vi "Testing.vi"() -> ()   [LabVIEW 2013]
panel:
  in  "Image Name":string="Test1"
  in  "File Name":string="Checkout1"
  out "Image":T1(plugin-control)
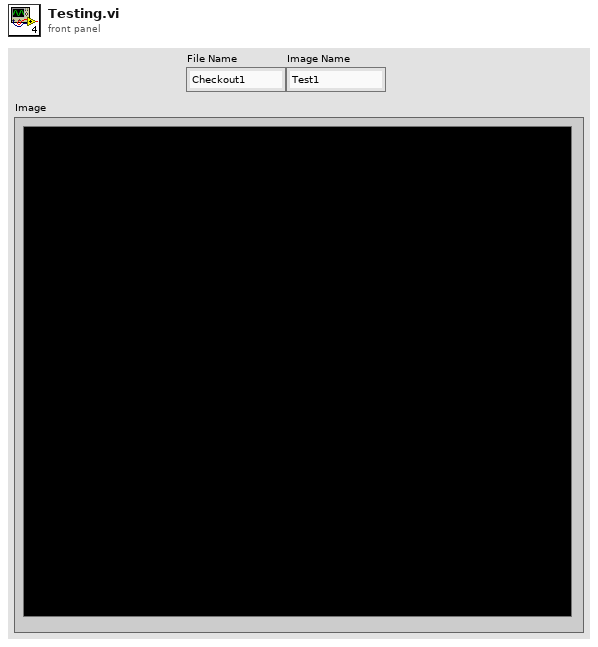
[diagram p1: front panel]
types:
  T1 = typedef "IMAQ Image.ctl" = refnum<image>
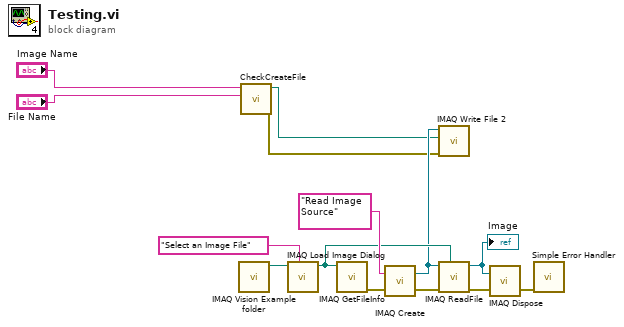
[diagram p0: block diagram]
diagram:
  n1 = call "IMAQ Vision Example folder.vi"() -> ("Example Image Path"=w11:path)  [unwired: 11 in]
  n2 = call "CheckCreateFile.vi"("File Name"="File Name", "Image Name"="Image Name") -> ("Error Out"=w1:errorcluster, "File Path"=w3:path)  [unwired: 8 in]
  n3 = call "IMAQ Load Image Dialog"("Prompt"="Select an Image File" ("prompt"), "Start Path"=w11) -> ("Path"=w8:path)  [unwired: 7 in, 2 out]
  n4 = call "IMAQ GetFileInfo"("File Path"=w8) -> ("error out"=w10:errorcluster)  [unwired: 4 in, 6 out]
  n5 = call "IMAQ Create"("Image Name"="Read Image Source", "error in (no error)"=w10) -> ("New Image"=w4:T1, "error out"=w13:errorcluster)  [unwired: 3 in]
  n6 = call-poly "IMAQ Write File 2"("error in (no error)"=w1, "File Path"=w3, "Image"=w4) -> ()  [unwired: 7 in, 2 out]
  n7 = call "IMAQ ReadFile"("File Path"=w8, "error in (no error)"=w13, "Image"=w4) -> ("error out"=w6:errorcluster, "Image Out"=w5:T1)  [unwired: 4 in, 3 out]
  "Image" <- w5
  n8 = call "IMAQ Dispose"("Image"=w5, "error in (no error)"=w6) -> ("error out"=w7:errorcluster)  [unwired: 4 in]
  n9 = call <vilib>:"Simple Error Handler.vi"("error in (no error)"=w7) -> ()  [unwired: 4 in, 5 out]
